vi "Start Open Loop Scan.vi"(8 "error in (no error)":errorcluster, 9 "Scan Settings":T1, 10 "Model in":refnum<class "Model.lvclass">, 11 "Wait For User Input State in":refnum<class "Wait For User Input State.lvclass">) -> (0 "error out":errorcluster, 2 "Model out":refnum<class "Model.lvclass">, 3 "Wait For User Input State out":refnum<class "Wait For User Input State.lvclass">)   [LabVIEW 2015]
uses:
  Model/Model/Model.lvclass
  Typedefs/State Types.ctl
  Typedefs/FAMT Typedefs.lvlib
  Wait For User Input State.lvclass
  Typedefs/Scan Settings.ctl
  Typedefs/Waveform Types.ctl
  Typedefs/Waveform Settings.ctl
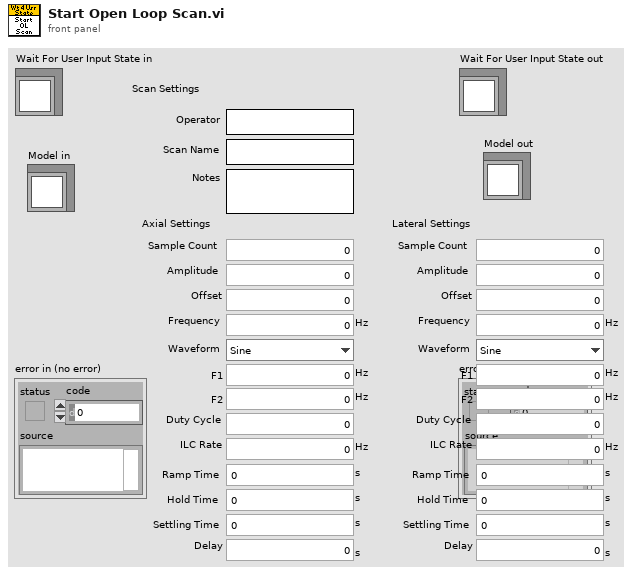
[diagram p1: front panel]
types:
  T1 = typedef "FAMT Typedefs.lvlib/Scan Settings.ctl" = cluster{"Operator":string, "Scan Name":string, "Notes":string, "Axial Settings":T2, "Lateral Settings":T2}
  T2 = typedef "FAMT Typedefs.lvlib/Waveform Settings.ctl" = cluster{"Sample Count":u32, "Amplitude":dbl, "Offset":dbl, "Frequency":dbl[unit], "Waveform":T3, "F1":dbl[unit], "F2":dbl[unit], "Duty Cycle":dbl, "ILC Rate":dbl[unit], "Ramp Time":dbl[unit], "Hold Time":dbl[unit], "Settling Time":dbl[unit], "Delay":dbl[unit]}
  T3 = typedef "FAMT Typedefs.lvlib/Waveform Types.ctl" = enum16{"Sine", "Triangle", "Square", "Sawtooth", "Chirp", "Gaussian", "Trapezoid"}
  T4 = typedef "FAMT Typedefs.lvlib/State Types.ctl" = enum16{"Offline State", "Fault State", "Standby State", "Disabled State", "Enabled State", "Wait For User Input State", "Perform Scan State"}
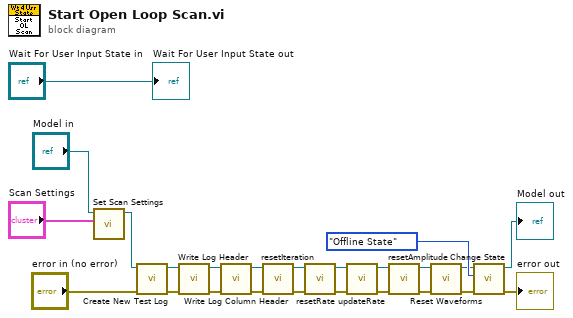
[diagram p0: block diagram]
diagram:
  n1 = call "Set Scan Settings.vi"("Scan Settings"="Scan Settings", "Model in"="Model in") -> ("Model out"=w16:refnum<class "Model.lvclass">)  [unwired: 9 in]
  n2 = call "Create New Test Log.vi"("error in (no error)"="error in (no error)", "Model in"=w16) -> ("error out"=w12:errorcluster, "Model out"=w15:refnum<class "Model.lvclass">)  [unwired: 8 in]
  n3 = call "Write Log Header.vi"("error in (no error)"=w12, "Model in"=w15) -> ("error out"=w11:errorcluster, "Model out"=w14:refnum<class "Model.lvclass">)  [unwired: 8 in]
  n4 = call "Write Log Column Header.vi"("error in (no error)"=w11, "Model in"=w14) -> ("error out"=w2:errorcluster, "Model out"=w1:refnum<class "Model.lvclass">)  [unwired: 8 in]
  n5 = call "resetIteration.vi"("error in (no error)"=w2, "Model in"=w1) -> ("error out"=w10:errorcluster, "Model out"=w19:refnum<class "Model.lvclass">)  [unwired: 8 in]
  n6 = call "resetRate.vi"("error in (no error)"=w10, "Model in"=w19) -> ("error out"=w9:errorcluster, "Model out"=w18:refnum<class "Model.lvclass">)  [unwired: 8 in]
  n7 = call "updateRate.vi"("error in (no error)"=w9, "Model in"=w18) -> ("error out"=w8:errorcluster, "Model out"=w17:refnum<class "Model.lvclass">)  [unwired: 8 in]
  n8 = call "resetAmplitude.vi"("error in (no error)"=w8, "Model in"=w17) -> ("error out"=w6:errorcluster, "Model out"=w3:refnum<class "Model.lvclass">)  [unwired: 8 in]
  n9 = call "Reset Waveforms.vi"("error in (no error)"=w6, "Model in"=w3) -> ("error out"=w5:errorcluster, "Model out"=w4:refnum<class "Model.lvclass">)  [unwired: 8 in]
  n10 = call "Change State.vi"("error in (no error)"=w5, "State Types"=State_Types."Offline State" ("State:"), "Model in"=w4) -> ("error out"=→"error out":errorcluster, "Model out"=→"Model out":refnum<class "Model.lvclass">)  [unwired: 7 in]
  "Wait For User Input State out" <- "Wait For User Input State in"
